vi "tsfifo_receive_lin_msgs.vi"(8 "错误输入（无错误）":errorcluster, 9 "Read message type":T1(ring)=enum."Receive&send messages", 10 "AIdxChn":i32, 11 "路径输入":path) -> (0 "错误输出":errorcluster, 1 "return":i32, 2 "ALINBuffer":T2[](array[typedef]), 3 "路径输出":path)   [LabVIEW 2014]
doc: "Function Introduction :\nList of received Lin messages\nCall location :\ninput parameter :\nALINBuffers: lin buffer\nALINBufferSize: lin buffer size\nAIdxChn: Channel Index\nAIncludeTx: Does it contain TX messages\nReturn value :\n0: Execution successful\nOther values: Failed"
uses:
  Typedef/TLibLIN.ctl
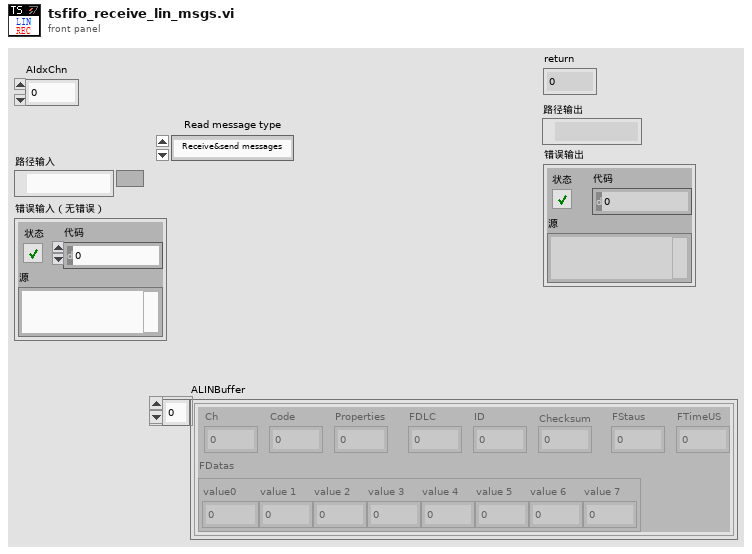
[diagram p1: front panel]
types:
  T1 = enum16{"Only read received messages", "Receive&send messages"}
  T2 = typedef "TLibLIN.ctl" = cluster{"Ch":u8, "Code":u8, "Properties":u8, "FDLC":u8, "ID":u8, "Checksum":u8, "FStaus":u8, "FTimeUS":u64, "FDatas":cluster{"value0":u8, "value 1":u8, "value 2":u8, "value 3":u8, "value 4":u8, "value 5":u8, "value 6":u8, "value 7":u8}}
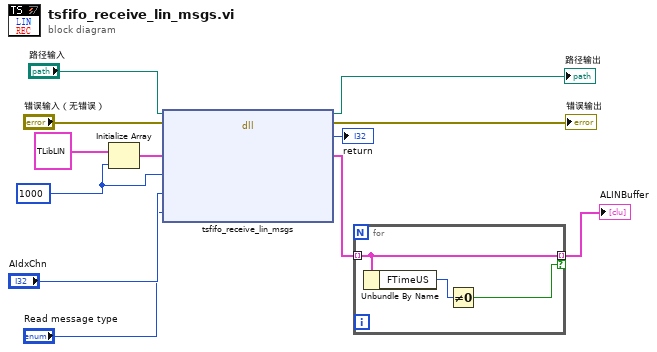
[diagram p0: block diagram]
diagram:
  w3 = 1000 ("维数大小")
  n1 = Initialize Array(T2 {"Ch"=0, "Code"=0, "Properties"=0, "FDLC"=0, "ID"=0, "Checksum"=0, "FStaus"=0, "FTimeUS"=0, "FDatas"={"value0"=0, "value 1"=0, "value 2"=0, "value 3"=0, "value 4"=0, "value 5"=0, "value 6"=0, "value 7"=0}} ("TLIBLIN"), w3) -> (w11:T2[])
  n2 = dll-call lib="D:/Program Files (x86)/TOSUN/TSMaster/Data/SDK/lib/x86/TSMaster.dll" fn="tsfifo_receive_lin_msgs"(path in="路径输入", error in="错误输入（无错误）", "ALINBuffer"=w11, "ALINBufferSize"=w3, "AIdxChn"="AIdxChn", "AIncludeTx"="Read message type") -> (path out=→"路径输出":path, error out=→"错误输出":errorcluster, "返回类型"=→"return":i32, "ALINBuffer"=w2:T2[])  [unwired: 4 in]
  n3 = for {
    tunnel: [w15] -> w5 mode=indexing if=w13
    tunnel: w2 -> [w15] mode=indexing
    n4 = Unbundle By Name(w15) -> ("FTimeUS"=w14:u64)
    n5 = Not Equal To 0?(x=w14) -> (x != 0?=w13:bool)
  }
  "ALINBuffer" <- w5
